vi "Resize Image.vi"(8 "error in (no error)":errorcluster, 11 "Save Image in":refnum<class "Save Image.lvclass">) -> (0 "error out":errorcluster, 3 "Save Image out":refnum<class "Save Image.lvclass">)   [LabVIEW 2018, in "Save Image.lvclass"]
uses:
  Save Image.lvclass
  <userlib>/gfitsio/cfitsio-bitpix.ctl
  Save Image.lvclass/Save Image.ctl
  Interface/Interface.lvclass/Interface.ctl
  Interface/Interface.lvclass
  <userlib>/gfitsio/gfitsio.lvlib
  Simulated_Header/Simulated_Header.lvclass
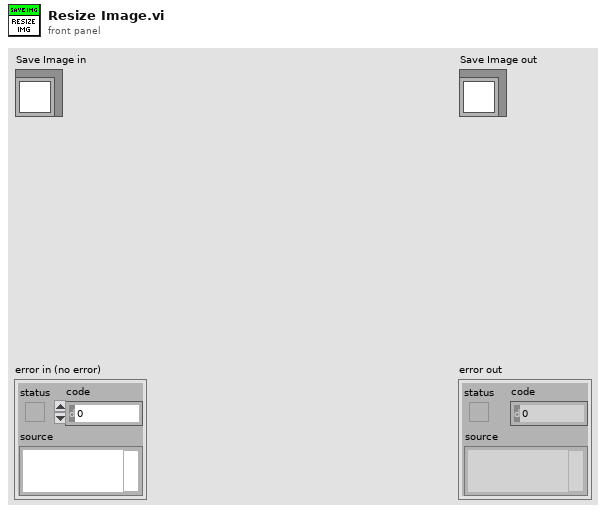
[diagram p1: front panel]
types:
  T1 = typedef "gfitsio.lvlib/cfitsio-bitpix.ctl" = i32
  T2 = cluster{"COOLER_POWER_STATUS":u16, "TEMP":i32, "EXPTIME":dbl, "#FRAMES":u32, "#CUBES":u32}
  T3 = typedef "Shutter_mode typedef.ctl" = enum16{"Auto", "Open", "Close", "N/A (3)", "Open FVB Series", "Open Any Series"}
  T4 = typedef "ReadMode_mode typedef.ctl" = enum16{"Full Vertical Binning", "Multi-Track", "Random-Track", "Single-Track", "Image"}
  T5 = typedef "AcquisitionMode_mode typedef.ctl" = enum16{"Reserved (0)", "Single Scan", "Accumulate", "Kinetics", "Fast Kinetics", "Run Till Abort", "Reserved (6)", "Reserved (7)", "Reserved (8)", "Time Delayed Integration"}
  T6 = cluster{"PREAMP":enum16{"Gain 1", "Gain 2"}, "READOUT_RATE":enum16{"30 MHz", "20 MHz", "10 MHz", "1 MHz"}, "EM_GAIN":u16, "VBIN":u16, "INITIAL_LINE":u16, "INITIAL_COLUMN":u16, "FINAL_LINE":u16, "FINAL_COLUMN":u16, "TRIGGER_MODE":enum16{"Internal", "External", "N/A", "N/A_1", "N/A_2", "N/A_3", "External Start"}, "HBIN":u16, "SHUTTER_TTL":enum16{"TTL Low", "TTL High"}, "SHUTTER_MODE":T3, "SHUTTER_OPENING_TIME":u16, "SHUTTER_CLOSING_TIME":u16, "VERTICAL_SHIFT_SPEED":u16, "READ_MODE":T4, "FRAME_TRANSFER":bool, "VERTICAL_CLOCK_VOLTAGE":enum16{"0", "+1", "+2", "+3", "+4"}, "ACQUISITION_MODE":T5, "AD_CHANNEL":u16, "EM_MODE":enum16{"Electron Multiplying", "Conventional"}}
  T7 = typedef "gfitsio.lvlib/gfitsio-refnum.ctl" = refnum<k1>
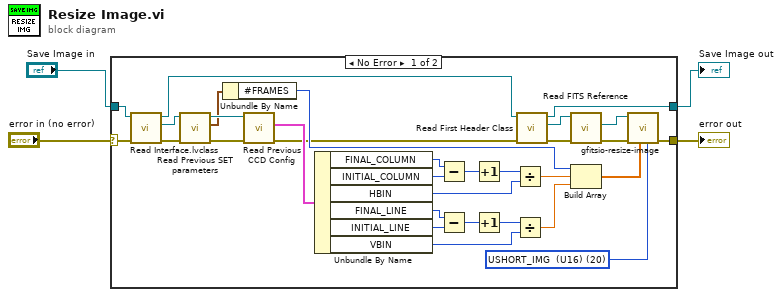
[diagram p0: block diagram]
diagram:
  n1 = case shown="No Error" "error in (no error)" {
    selector: "error in (no error)" -> [w10 w37]
    tunnel: [w16 w37] -> w3
    tunnel: [w5 w36] -> w1
    tunnel: "Save Image in" -> [w11 w36]
    frame No Error {
      w35 = T1 20 items=["<invalid type>"=0, "BYTE_IMG  (U8)"=8, "SHORT_IMG  (I16)"=16, "USHORT_IMG  (U16)"=20, "LONG_IMG  (I32)"=32, "ULONG_IMG  (U32)"=40, "FLOAT_IMG  (SGL)"=-32, "DOUBLE_IMG  (DBL)"=-64] ("image data type")
      n2 = call "Read Interface.lvclass.vi"("error in (no error)"=w10, "Save Image in"=w11) -> ("error out"=w9:errorcluster, "Interface.lvclass"=w8:refnum<class "Interface.lvclass">, "Save Image out"=w7:refnum<class "Save Image.lvclass">)  [unwired: 7 in]
      n3 = call "Read Previous SET parameters.vi"("error in (no error)"=w9, "Interface in"=w8) -> ("error out"=w27:errorcluster, "Previous SET parameters"=w25:T2, "Interface out"=w26:refnum<class "Interface.lvclass">)  [unwired: 7 in]
      n4 = Unbundle By Name(w25) -> ("#FRAMES"=w24:u32)
      n5 = call "Read Previous CCD Config.vi"("error in (no error)"=w27, "Interface in"=w26) -> ("error out"=w6:errorcluster, "Previous CCD Config"=w34:T6)  [unwired: 7 in, 1 out]
      n6 = Unbundle By Name(w34) -> ("FINAL_COLUMN"=w33:u16, "INITIAL_COLUMN"=w32:u16, "HBIN"=w29:u16, "FINAL_LINE"=w31:u16, "INITIAL_LINE"=w30:u16, "VBIN"=w28:u16)
      n7 = Subtract(x=w33, y=w32) -> (x-y=w20:u16)
      n8 = Subtract(x=w31, y=w30) -> (x-y=w18:u16)
      n9 = Increment(x=w20) -> (x+1=w19:u16)
      n10 = Increment(x=w18) -> (x+1=w17:u16)
      n11 = Divide(x=w19, y=w29) -> (x/y=w23:dbl)
      n12 = Divide(x=w17, y=w28) -> (x/y=w22:dbl)
      n13 = call "Read First Header Class.vi"("error in (no error)"=w6, "Save Image in"=w7) -> ("error out"=w14:errorcluster, "Simulated_Header.lvclass"=w15:refnum<class "Simulated_Header.lvclass">, "Save Image out"=w5:refnum<class "Save Image.lvclass">)  [unwired: 7 in]
      n14 = call "Read FITS Reference.vi"("error in (no error)"=w14, "Simulated_Header in"=w15) -> ("error out"=w13:errorcluster, "gfits refnum"=w12:T7)  [unwired: 7 in, 1 out]
      n15 = Build Array(w24, w23, w22) -> (w21:dbl[])
      n16 = call <userlib>:"gfitsio-resize-image.vi"("image data type"=w35, "naxes"=w21, "error in (no error)"=w13, "gfits refnum"=w12) -> ("error out"=w16:errorcluster)  [unwired: 6 in, 1 out]
    }
    frame Error {
    }
  }
  "error out" <- w3
  "Save Image out" <- w1
